vi "Read HDI Fiducials.vi"(8 "error in":errorcluster, 9 "Slot":u32, 11 "CameraTool in":refnum<class "CameraTool Class.lvclass">) -> (0 "error out":errorcluster, 3 "CameraTool out":refnum<class "CameraTool Class.lvclass">)   [LabVIEW 2011, in "CameraTool Class.lvclass"]
uses:
  CameraTool Class.lvclass
  WorkTable Class/WorkTable Class.lvclass
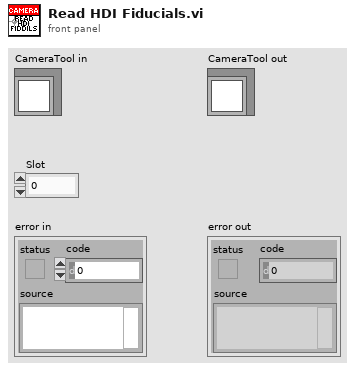
[diagram p1: front panel]
types:
  T1 = cluster{"Fiducial Type":string, "Selection Criteria":enum16{"Single", "Top", "Bottom"}}
  T2 = typedef "Worktable_HDI Slot.ctl" = cluster{"HDI Assembly State":enum16{"Empty", "Populated"}, "HDI Type":enum16{"HDI", "Polyimide"}, "Vacuum Channel":u32, "Location/Orientation":T3}
  T3 = typedef "Position_Orientation.ctl" = cluster{"Center":refnum<class "Vec3d Class.lvclass">, "Orientation":refnum<class "Orient3d Class.lvclass">}
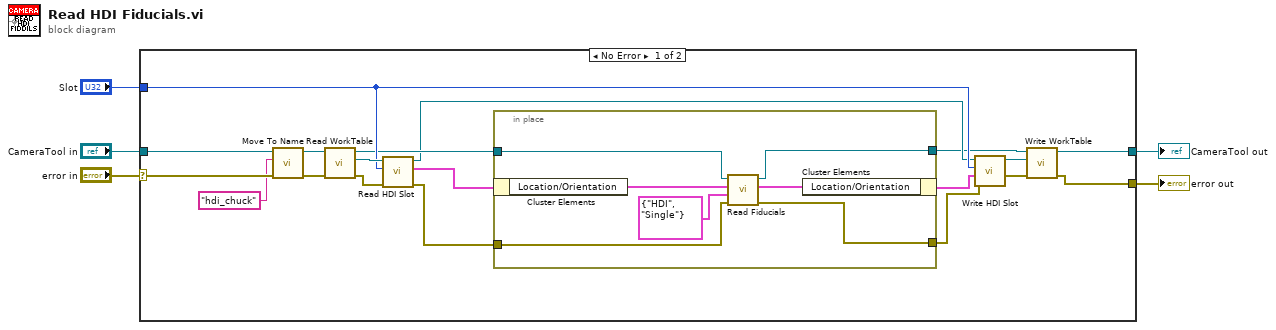
[diagram p0: block diagram]
diagram:
  n1 = case shown="No Error" "error in" {
    selector: "error in" -> [w15 w33]
    tunnel: [w16 w33] -> w1
    tunnel: [w17 w32] -> w2
    tunnel: "CameraTool in" -> [w18 w32]
    tunnel: "Slot" -> [w13 _]
    frame No Error {
      n2 = call-dynamic "Move To Name.vi"("error in"=w15, "Destination Name"="hdi_chuck" ("format string"), "Gantry in"=w18) -> ("error out"=w24:errorcluster, "Gantry out"=w23:refnum<class "CameraTool Class.lvclass">)  [unwired: 7 in]
      n3 = call-dynamic "Read WorkTable.vi"("error in"=w24, "Gantry Class in"=w23) -> ("error out"=w21:errorcluster, "WorkTable Class.lvclass"=w22:refnum<class "WorkTable Class.lvclass">, "Gantry Class out"=w11:refnum<class "CameraTool Class.lvclass">)  [unwired: 7 in]
      n4 = call-dynamic "Read HDI Slot.vi"("error in"=w21, "HDI Slot Number"=w13, "WorkTable in"=w22) -> ("error out"=w12:errorcluster, "HDI Slot"=w10:T2, "WorkTable out"=w8:refnum<class "WorkTable Class.lvclass">)  [unwired: 6 in]
      n5 = in-place {
        in-place-border: w12 -> [w27]
        in-place-border: w11 -> [w29]
        in-place-border: [w28] -> w7
        in-place-border: [w26] -> w6
        n6 = in-place-cluster #1(w10) -> ("Location/Orientation"=w31:T3)
        n7 = call-dynamic "Read Fiducials.vi"("error in"=w27, "Fiducial Acquisition Parameters"=T1 {"Fiducial Type"="HDI", "Selection Criteria"=enum."Single"}, "Location/Orientation in"=w31, "CameraTool in"=w29) -> ("error out"=w26:errorcluster, "Location/Orientation out"=w30:T3, "CameraTool out"=w28:refnum<class "CameraTool Class.lvclass">)  [unwired: 5 in]
        n8 = in-place-cluster #1("Location/Orientation"=w30) -> (w9:T2)
      }
      n9 = call-dynamic "Write HDI Slot.vi"("error in"=w6, "HDI Slot"=w9, "HDI Slot Number"=w13, "WorkTable in"=w8) -> ("error out"=w19:errorcluster, "WorkTable out"=w20:refnum<class "WorkTable Class.lvclass">)  [unwired: 6 in]
      n10 = call-dynamic "Write WorkTable.vi"("error in (no error)"=w19, "WorkTable Class.lvclass"=w20, "Gantry Class in"=w7) -> ("error out"=w16:errorcluster, "Gantry Class out"=w17:refnum<class "CameraTool Class.lvclass">)  [unwired: 7 in]
    }
    frame Error {
    }
  }
  "error out" <- w1
  "CameraTool out" <- w2
